vi "SuperAuton-CanGrab.vi"(9 "TimeToPull":dbl) -> (2 "Success?":bool)   [LabVIEW 2014]
uses:
  Robot Global Data.vi
  <vilib>/Rock Robotics/WPI/RobotDrive/WPI_RobotDriveGetSetRefNum.vi
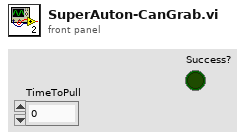
[diagram p1: front panel]
types:
  T1 = typedef "WPI_RobotDriveDevRef.ctl" = cluster{"DevStatus":errorcluster, "Motors[]":T2[], "Square Inputs":bool, "Max Output":dbl}
  T2 = typedef "WPI_MotorControlDeviceRef.ctl" = cluster{"DeviceStatus":errorcluster, "Type":T3, "PWM":cluster{"Controller":T4, "PWM Channel":T5, "DeadBand":T6}, "CAN":cluster{"Device Number":u8, "Control Mode":T7, "Semaphore":T8, "Max Vout":dbl, "TalonSRX Control Mode":T9}, "Invert":bool, "TransformRef":T10, "InvTransformRef":T10}
  T3 = typedef "WPI_MotorControlType.ctl" = enum16{"PWM", "CAN", "CANTalonSRX"}
  T4 = typedef "FPGA_TypedefDigitalModule.ctl" = enum16{"Controller 1"}
  T5 = typedef "FPGA_DIOPWMChannel.ctl" = enum8{"PWM 0", "PWM 1", "PWM 2", "PWM 3", "PWM 4", "PWM 5", "PWM 6", "PWM 7", "PWM 8", "PWM 9", "PWM MXP 0", "PWM MXP 1", "PWM MXP 2", "PWM MXP 3", "PWM MXP 4", "PWM MXP 5", "PWM MXP 6", "PWM MXP 7", "PWM MXP 8", "PWM MXP 9", "Invalid"}
  T6 = typedef "WPI_PWMDeadband.ctl" = cluster{"Name":string, "maxPositivePwm":i32, "minPositivePwm":i32, "centerPwm":i32, "maxNegativePwm":i32, "minNegativePwm":i32, "angularRange":u16}
  T7 = typedef "WPI_CANJaguar_ControlMode.ctl" = enum8{"Percent VBus", "Current", "Speed", "Position", "Voltage"}
  T8 = typedef "Semaphore RefNum" = refnum<k1>
  T9 = typedef "WPI_CANTalonSRX_APIControlMode.ctl" = enum8{"Percent VBus", "Speed", "Position", "Slave", "Unchanged / Invalid"}
  T10 = typedef "WPI_PWMTransform_ConPane.ctl" = refnum<vi>
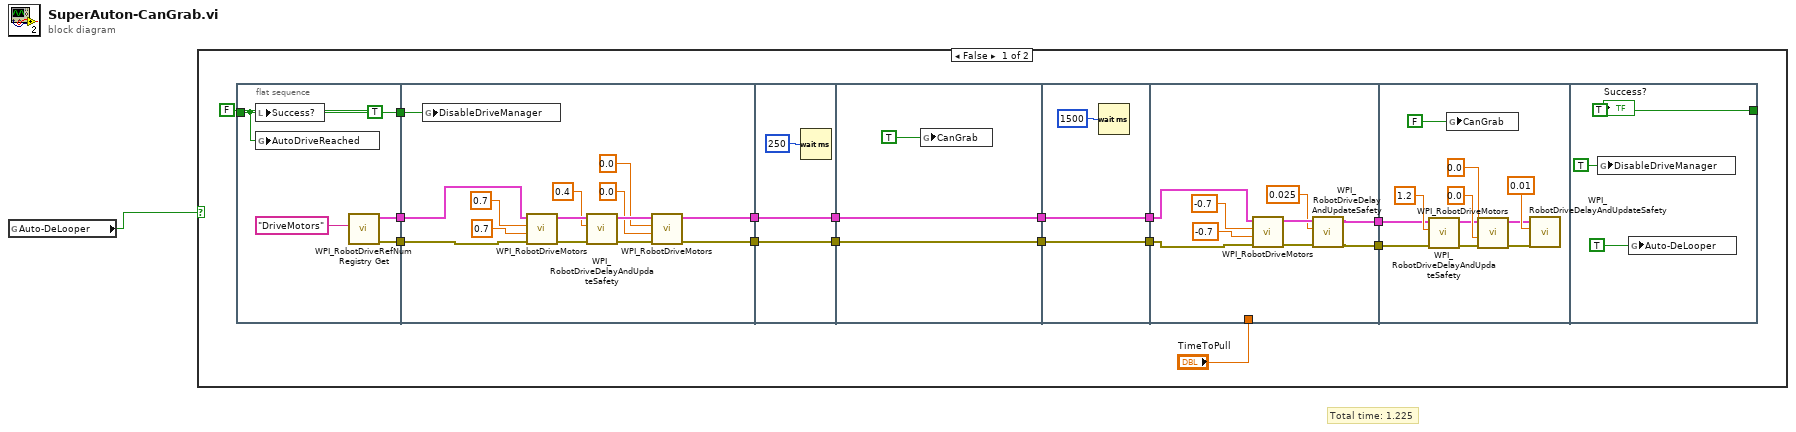
[diagram p0: block diagram]
diagram:
  # "Total time: 1.225"
  n1 = global read "Robot Global Data.vi" "Auto-DeLooper"() -> (w1:bool)
  n2 = case shown="False" w1 {
    frame False {
      n3 = flat-sequence {
        tunnel: FALSE ("Success?") -> [w22]
        tunnel: [TRUE ("Success?")] -> w15
        tunnel: [w19] -> w16
        tunnel: [w18] -> w17
        tunnel: w17 -> [w34]
        tunnel: w16 -> [w35]
        tunnel: w15 -> [w36]
        tunnel: [w33] -> w14
        tunnel: [w32] -> w13
        tunnel: w14 -> [w39]
        tunnel: [w39] -> w12
        tunnel: w13 -> [w38]
        tunnel: [w38] -> w11
        tunnel: w12 -> [w41]
        tunnel: w11 -> [w40]
        tunnel: [w41] -> w10
        tunnel: [w40] -> w9
        tunnel: [w44] -> w8
        tunnel: w10 -> [w44]
        tunnel: [w43] -> w7
        tunnel: w9 -> [w43]
        tunnel: "TimeToPull" -> [_]
        tunnel: w8 -> [w48]
        tunnel: w7 -> [w49]
        tunnel: [w47] -> w6
        tunnel: [w46] -> w5
        tunnel: w6 -> [w59]
        tunnel: w5 -> [w56]
        tunnel: [TRUE ("Success?")] -> w4
        frame #0 {
          n4 = local write "Success?"(w22) -> ()
          n5 = global write "Robot Global Data.vi" "AutoDriveReached"(w22) -> ()
          n6 = call <vilib>:"WPI_RobotDriveRefNum Registry Get.vi"("refnum name"="DriveMotors") -> ("error out"=w18:errorcluster, "RobotDriveDevRef"=w19:T1)  [unwired: 9 in]
        }
        frame #1 {
          n7 = global write "Robot Global Data.vi" "DisableDriveManager"(w36) -> ()
          n8 = call <vilib>:"WPI_RobotDriveMotors.vi"("error in (no error)"=w34, "RightSpeed"=0.7 ("Y axis value"), "LeftSpeed"=0.7 ("X axis value"), "RobotDriveDevRef"=w35) -> ("error out"=w28:errorcluster, "RobotDriveDevRef"=w29:T1)  [unwired: 5 in, 1 out]
          n9 = call <vilib>:"WPI_RobotDriveDelayAndUpdateSafety.vi"("error in (no error)"=w28, "Delay (s)"=0.4, "RobotDriveDevRef"=w29) -> ("error out"=w25:errorcluster, "RobotDriveDevRef 2"=w26:T1)  [unwired: 7 in]
          n10 = call <vilib>:"WPI_RobotDriveMotors.vi"("error in (no error)"=w25, "RightSpeed"=0.0 ("Y axis value"), "LeftSpeed"=0.0 ("X axis value"), "RobotDriveDevRef"=w26) -> ("error out"=w32:errorcluster, "RobotDriveDevRef"=w33:T1)  [unwired: 5 in, 1 out]
        }
        frame #2 {
          n11 = Wait (ms)(milliseconds to wait=u32 250) -> ()  [unwired: 1 out]
        }
        frame #3 {
          n12 = global write "Robot Global Data.vi" "CanGrab"(TRUE) -> ()
        }
        frame #4 {
          n13 = Wait (ms)(milliseconds to wait=u32 1500) -> ()  [unwired: 1 out]
        }
        frame #5 {
          n14 = call <vilib>:"WPI_RobotDriveMotors.vi"("error in (no error)"=w49, "RightSpeed"=-0.7 ("Y axis value"), "LeftSpeed"=-0.7 ("X axis value"), "RobotDriveDevRef"=w48) -> ("error out"=w51:errorcluster, "RobotDriveDevRef"=w52:T1)  [unwired: 5 in, 1 out]
          n15 = call <vilib>:"WPI_RobotDriveDelayAndUpdateSafety.vi"("error in (no error)"=w51, "Delay (s)"=0.025, "RobotDriveDevRef"=w52) -> ("error out"=w46:errorcluster, "RobotDriveDevRef 2"=w47:T1)  [unwired: 7 in]
        }
        frame #6 {
          n16 = call <vilib>:"WPI_RobotDriveDelayAndUpdateSafety.vi"("error in (no error)"=w56, "Delay (s)"=1.2, "RobotDriveDevRef"=w59) -> ("error out"=w57:errorcluster, "RobotDriveDevRef 2"=w58:T1)  [unwired: 7 in]
          n17 = global write "Robot Global Data.vi" "CanGrab"(FALSE) -> ()
          n18 = call <vilib>:"WPI_RobotDriveMotors.vi"("error in (no error)"=w57, "RightSpeed"=0.0 ("Y axis value"), "LeftSpeed"=0.0 ("X axis value"), "RobotDriveDevRef"=w58) -> ("error out"=w63:errorcluster, "RobotDriveDevRef"=w64:T1)  [unwired: 5 in, 1 out]
          n19 = call <vilib>:"WPI_RobotDriveDelayAndUpdateSafety.vi"("error in (no error)"=w63, "Delay (s)"=0.01, "RobotDriveDevRef"=w64) -> ()  [unwired: 7 in, 2 out]
        }
        frame #7 {
          n20 = global write "Robot Global Data.vi" "DisableDriveManager"(TRUE ("DisableDriveManager")) -> ()
          n21 = global write "Robot Global Data.vi" "Auto-DeLooper"(TRUE ("DisableDriveManager")) -> ()
        }
      }
      "Success?" <- w4
    }
    frame True {
    }
  }
